vi "MakeExample.vi"(8 "error in (no error)":errorcluster, 9 "TriggerRefractoryPeriod (Frames)":i32, 10 "StimulusObject Parameters":variant, 11 "StimOnHeadBends in":refnum<class "StimOnHeadBends.lvclass">) -> (0 "error out":errorcluster, 3 "StimOnHeadBends out":refnum<class "StimOnHeadBends.lvclass">)   [LabVIEW 2019, in "StimOnHeadBends.lvclass"]
uses:
  StimOnHeadBends.lvclass
  StimOnHeadBendsInputCluster.ctl
  StimOnHeadBends.lvclass/StimOnHeadBends.ctl
  ParametersGlobal.vi
  StimulusObject.lvclass
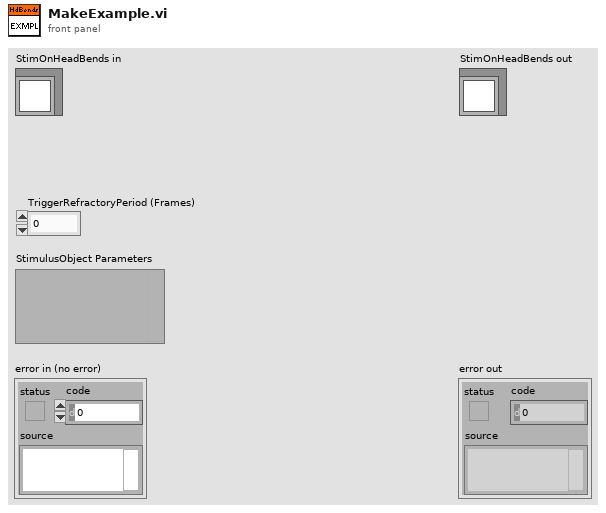
[diagram p1: front panel]
types:
  T1 = typedef "StimOnHeadBends.lvclass/StimOnHeadBendsInputCluster.ctl" = cluster{"Constant Intensity (uW/mm^2, negative is blue)":sgl, "dot radius (mm)":sgl, "Intensities (uW/mm^2, negative is blue)":sgl[], "Durations (s)":sgl[], "Inter trigger interval (s)":dbl, "Ellipse Ratio Trigger Point":sgl, "Wait time after reversal is detected (s)":dbl}
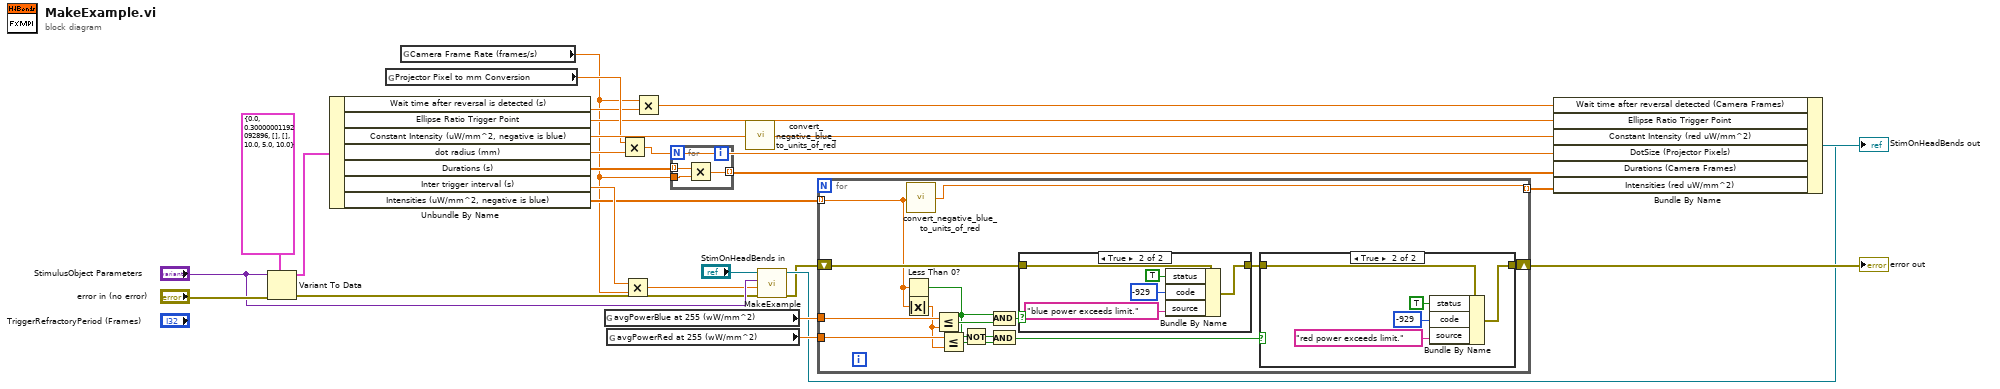
[diagram p0: block diagram]
diagram:
  n1 = Variant To Data(error in="error in (no error)", type=T1 {"Constant Intensity (uW/mm^2, negative is blue)"=0.0, "dot radius (mm)"=0.3, "Intensities (uW/mm^2, negative is blue)"=[], "Durations (s)"=[], "Inter trigger interval (s)"=10.0, "Ellipse Ratio Trigger Point"=5.0, "Wait time after reversal is detected (s)"=10.0} ("StimOnHeadBendsInputCluster"), Variant="StimulusObject Parameters") -> (data=w27:T1, error out=w7:errorcluster)
  n2 = Unbundle By Name(w27) -> ("Wait time after reversal is detected (s)"=w3:dbl, "Ellipse Ratio Trigger Point"=w14:sgl, "Constant Intensity (uW/mm^2, negative is blue)"=w25:sgl, "dot radius (mm)"=w23:sgl, "Durations (s)"=w20:sgl[], "Inter trigger interval (s)"=w26:dbl, "Intensities (uW/mm^2, negative is blue)"=w18:sgl[])
  n3 = global read "ParametersGlobal.vi" "Projector Pixel to mm Conversion"() -> (w22:sgl)
  n4 = global read "ParametersGlobal.vi" "Camera Frame Rate (frames/s)"() -> (w2:sgl)
  n5 = global read "ParametersGlobal.vi" "avgPowerBlue at 255 (wW/mm^2)"() -> (w17:sgl)
  n6 = global read "ParametersGlobal.vi" "avgPowerRed at 255 (wW/mm^2)"() -> (w16:sgl)
  n7 = Multiply(x=w22, y=w23) -> (x*y=w21:sgl)
  n8 = Multiply(x=w26, y=w2) -> (x*y=w8:dbl)
  n9 = Multiply(x=w2, y=w3) -> (x*y=w1:dbl)
  n10 = for {
    tunnel: w20 -> [w30] mode=indexing
    tunnel: w2 -> [w29]
    tunnel: [w28] -> w19 mode=indexing
    n11 = Multiply(x=w30, y=w29) -> (x*y=w28:sgl)
  }
  n12 = call "convert_negative_blue_to_units_of_red.vi"("Intensity in units of red (positive) and blue (negative)"=w25) -> ("Intensity in units of red (positive and negative)"=w24:sgl)
  n13 = call-parent "MakeExample.vi"("error in (no error)"=w7, "TriggerRefractoryPeriod (Frames)"=w8, "StimulusObject Parameters"="StimulusObject Parameters", "StimulusObject in"="StimOnHeadBends in") -> ("error out"=w5:errorcluster, "StimulusObject out"=w6:refnum<class "StimOnHeadBends.lvclass">)  [unwired: 6 in]
  n14 = for {
    tunnel: w18 -> [w38] mode=indexing
    shift-right: [w42] -> w11
    shift-left: w5 -> [w43]
    tunnel: w17 -> [w41]
    tunnel: w16 -> [w40]
    tunnel: [w39] -> w15 mode=indexing
    n15 = Less Than 0?(x=w38) -> (x < 0?=w31:bool)
    n16 = Absolute Value(x=w38) -> (abs(x)=w37:sgl)
    n17 = call "convert_negative_blue_to_units_of_red.vi"("Intensity in units of red (positive) and blue (negative)"=w38) -> ("Intensity in units of red (positive and negative)"=w39:sgl)
    n18 = Less Or Equal?(x=w41, y=w37) -> (x <= y?=w36:bool)
    n19 = Less Or Equal?(x=w40, y=w37) -> (x <= y?=w33:bool)
    n20 = Not(x=w31) -> (.not. x?=w32:bool)
    n21 = And(x=w31, y=w36) -> (x .and. y?=w35:bool)
    n22 = And(x=w32, y=w33) -> (x .and. y?=w34:bool)
    n23 = case shown="True" w35 {
      tunnel: w43 -> [w51 w56]
      tunnel: [w51 w55] -> w44
      frame False {
      }
      frame True {
        n24 = Bundle By Name(cluster=w56, "status"=TRUE, "code"=-929, "source"="blue power exceeds limit.") -> (w55:errorcluster)
      }
    }
    n25 = case shown="True" w34 {
      tunnel: w44 -> [w45 w50]
      tunnel: [w45 w49] -> w42
      frame False {
      }
      frame True {
        n26 = Bundle By Name(cluster=w50, "status"=TRUE, "code"=-929, "source"="red power exceeds limit.") -> (w49:errorcluster)
      }
    }
  }
  "error out" <- w11
  n27 = Bundle By Name(cluster=w6, "Wait time after reversal detected (Camera Frames)"=w1, "Ellipse Ratio Trigger Point"=w14, "Constant Intensity (red uW/mm^2)"=w24, "DotSize (Projector Pixels)"=w21, "Durations (Camera Frames)"=w19, "Intensities (red uW/mm^2)"=w15) -> (→"StimOnHeadBends out":refnum<class "StimOnHeadBends.lvclass">)
